vi "Z Aux Read U File.vi"(8 "error in (no error)":errorcluster caption="错误输入（无错误）", 9 "pinum":i32, 10 "pVarlist":sgl, 11 "sFilename":string) -> (0 "error out":errorcluster caption="错误输出", 1 "pinum out":i32, 2 "pVarlist out":sgl, 3 "function return":i32)   [LabVIEW 2015, in "zauxdll.lvlib"]
doc: "int32 __stdcall ZAux_ReadUFile(const char *sFilename, float *pVarlist, int* pinum);"
uses:
  zauxdll.lvlib
  zauxdll.dll
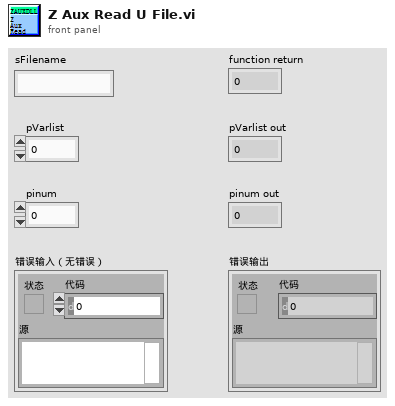
[diagram p1: front panel]
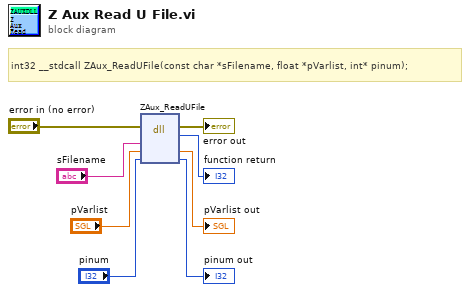
[diagram p0: block diagram]
diagram:
  # "int32 __stdcall ZAux_ReadUFile(const char *sFilename, float *pVarlist, int* pinum);"
  n1 = dll-call lib="C:/Users/VIC/Desktop/GOGORO_Oringnal - Panasonic/system/LLB/zmotion/zaux/zauxdll.*" fn="ZAux_ReadUFile"(error in="error in (no error)", "sFilename"="sFilename", "pVarlist"="pVarlist", "pinum"="pinum") -> (error out=→"error out":errorcluster, →"function return":i32, "pVarlist"=→"pVarlist out":sgl, "pinum"=→"pinum out":i32)  [unwired: 3 in, 1 out]
